vi "GDSLvIcon_UpdateLibraryLayers.vi"(0 "Library Refnum in":refnum<vi>, 1 "FrameColor":u32(colorbox), 2 "FrameThickness(1)":u32=1, 3 "HeaderIconIn":u8[][](array[numeric]) format="%x", 5 "error in (no error)":errorcluster, 11 "0px Splitter(False)":bool) -> (14 "Library Refnum out":refnum<vi>, 19 "error out":errorcluster)   [LabVIEW 2020]
uses:
  <vilib>/LabVIEW Icon API/API_User Layer Data.ctl
  <vilib>/Utility/miscctls.llb/LVPoint32TypeDef.ctl
  <vilib>/picture/picture.llb/imagedata.ctl
  <vilib>/LabVIEW Icon API/lv_icon/Classes/Icon/Icon.lvclass
  <vilib>/LabVIEW Icon API/lv_icon/lv_icon.lvlib
  <vilib>/LabVIEW Icon API/LabVIEW Icon API.lvlib
panel:
  out "LargeIconPictureOut(x6)":picture
  out "HeaderIcon":u8[][](array[numeric]) format="%x"
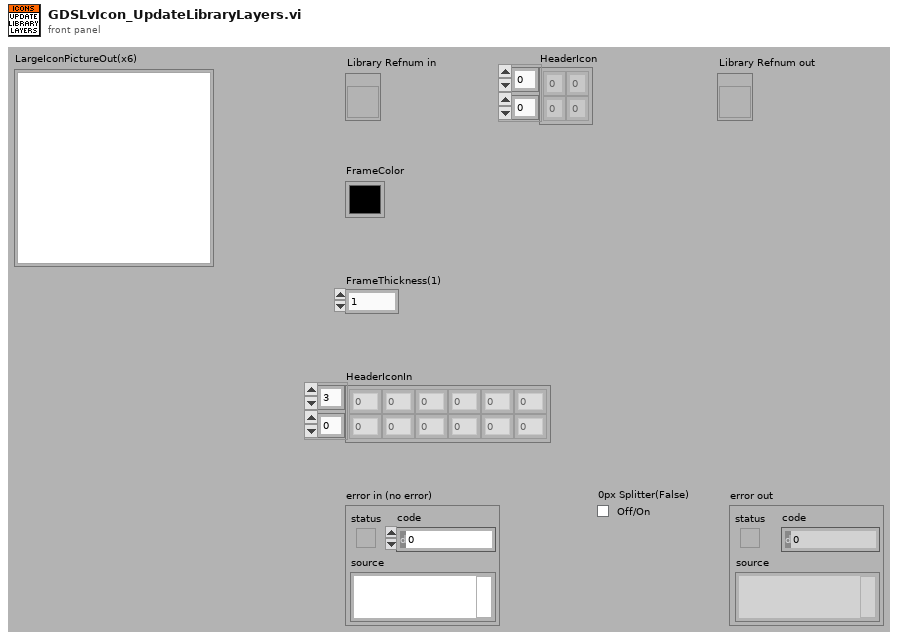
[diagram p1: front panel]
types:
  T1 = typedef "LabVIEW Icon API.lvlib/API_User Layer Data.ctl" = cluster{"Layer name":string, "Origin":T2, "Icon image data":T3}
  T2 = typedef "LVPoint32TypeDef.ctl" = cluster{"Horizontal":i32, "Vertical":i32}
  T3 = typedef "imagedata.ctl" = cluster{"image type":i32, "image depth":i32, "image":u8[], "mask":u8[], "colors":u32[], "Rectangle":cluster{"left":i16, "top":i16, "right":i16, "bottom":i16}}
  T4 = typedef "LabVIEW Icon Stored Information.ctl" = cluster{"Text Visible?":bool, "Text Opacity":u8, "Templ Visible?":bool, "Templ Opacity":u8, "Relative Path from 1 to 2":path, "Image":picture, "All User Layers":refnum<class "Layer.lvclass">[], "Body Text":T5}
  T5 = typedef "BodyText.ctl" = cluster{"Line 1 text":string, "Line 2 text":string, "Line 3 text":string, "Line 4 text":string, "Line 1 color":u32, "Line 2 color":u32, "Line 3 color":u32, "Line 4 color":u32, "Body Text Spec":cluster{"Font":T6, "Alignment":T7, "Size":u8}, "Center text vertically":bool, "Capitalize Text":bool}
  T6 = typedef "Font.ctl" = string
  T7 = typedef "Alignment.ctl" = u16
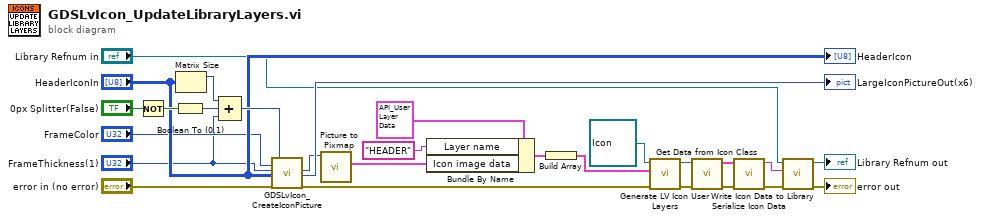
[diagram p0: block diagram]
diagram:
  n1 = Not(x="0px Splitter(False)") -> (.not. x?=w26:bool)
  n2 = Boolean To (0,1)(Boolean=w26) -> (0, 1=w25:i16)
  n3 = Matrix Size(0:"HeaderIconIn") -> (1:w27:i32)  [unwired: 1 out]
  n4 = Compound Arithmetic op=ADD(w27, w25, "FrameThickness(1)") -> (w24:u32)
  n5 = call <resource>:"GDSLvIcon_CreateIconPicture.vi"("FrameColor"="FrameColor", "FrameThickness(1)"="FrameThickness(1)", "HeaderIconIn"="HeaderIconIn", "error in (no error)"="error in (no error)", "ImageRows(32)"=w24) -> ("IconPictureOut"=w14:picture, "LargeIconPictureOut(x6)"=→"LargeIconPictureOut(x6)":picture, "error out"=w3:errorcluster)  [unwired: 9 in, 3 out]
  n6 = call <vilib>:"Picture to Pixmap.vi"("picture"=w14) -> ("image data"=w19:T3)  [unwired: 9 in, 1 out]
  n7 = Bundle By Name(cluster=T1 {"Layer name"="", "Origin"={"Horizontal"=0, "Vertical"=0}, "Icon image data"={"image type"=0, "image depth"=0, "image"=[], "mask"=[], "colors"=[], "Rectangle"={"left"=0, "top"=0, "right"=0, "bottom"=0}}} ("User layer"), "Layer name"="HEADER", "Icon image data"=w19) -> (w16:T1)
  n8 = Build Array(w16) -> (w15:T1[])
  n9 = call <vilib>:"Generate LV Icon User Layers.vi"("error in (no error)"=w3, "User layers"=w15, "Icon in"=refnum<class "Icon.lvclass"> refnum) -> ("error out"=w4:errorcluster, "Icon out"=w21:refnum<class "Icon.lvclass">)  [unwired: 7 in]
  n10 = call <vilib>:"Get Data from Icon Class.vi"("error in (no error)"=w4, "Icon in"=w21) -> ("error out"=w12:errorcluster, "Icon data"=w23:T4)  [unwired: 6 in, 2 out]
  n11 = call <vilib>:"Serialize Icon Data.vi"("error in"=w12, "Icon data"=w23) -> ("error out"=w13:errorcluster, "data string"=w22:string)  [unwired: 8 in]
  n12 = call <vilib>:"Write Icon Data to Library.vi"("error in (no error)"=w13, "Data"=w22, "Library Ref in"="Library Refnum in") -> ("error out"=→"error out":errorcluster, "Library Ref out"=→"Library Refnum out":refnum<vi>)  [unwired: 7 in]
  "HeaderIcon" <- "HeaderIconIn"
